vi "05_EventStructure5.vi"() -> ()   [LabVIEW 2019]
panel:
  in  "Enable Timeout":bool
  out "Numeric":i32
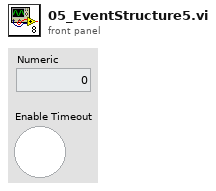
[diagram p1: front panel]
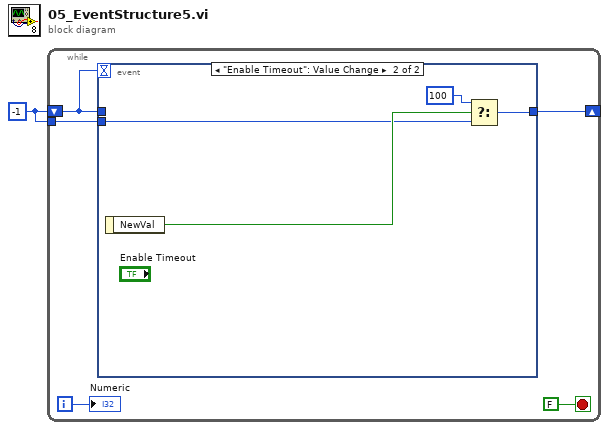
[diagram p0: block diagram]
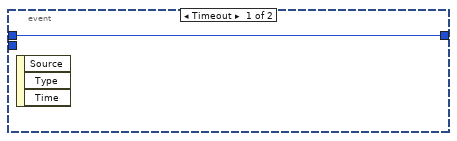
[diagram p2: hidden frame]
diagram:
  w1 = -1 ("t")
  n1 = while {
    shift-right: [w5] -> _
    shift-left: w1 -> [w3]
    tunnel: w1 -> [w4]
    i -> [w6]
    stop <- FALSE stop-if-true
    n2 = event shown="[1] \"Enable Timeout\": Value Change" {
      selector: _ -> [_ _]
      dyn-events: _ -> [_ _]
      timeout: w3 -> [_ _]
      tunnel: [w7 w11] -> w5
      tunnel: w3 -> [w7 _]
      tunnel: w4 -> [_ w8]
      event Timeout {
        n3 = event-data() -> ()  [unwired: 1 in, 3 out]
      }
      event "Enable Timeout": Value Change {
        n4 = event-data() -> ("NewVal"=w10:bool)  [unwired: 1 in]
        n5 = Select(t=100, s=w10, f=w8) -> (s? t:f=w11:i32)
      }
    }
    "Numeric" <- w6
  }
